vi "Read INI File.vi"(6 "Key":string, 8 "error in (no error)":errorcluster, 11 "Terminal Message in":refnum<class "Terminal Message.lvclass">) -> (0 "error out":errorcluster, 3 "Terminal Message out":refnum<class "Terminal Message.lvclass">, 4 "Message":string)   [LabVIEW 2016, in "CLD Exam - ATM.lvlib" / "Terminal Message.lvclass"]
uses:
  Terminal Message.lvclass
  Terminal Message.lvclass/Terminal Message.ctl
  <vilib>/Utility/config.llb/Read Key (String).vi
  <vilib>/Utility/config.llb/NI_LVConfig.lvlib
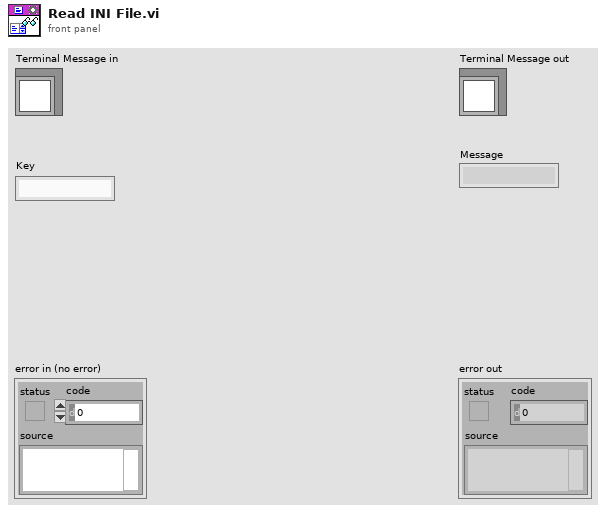
[diagram p1: front panel]
types:
  T1 = typedef "NI_LVConfig.lvlib/Config Data RefNum.ctl" = refnum<k1>
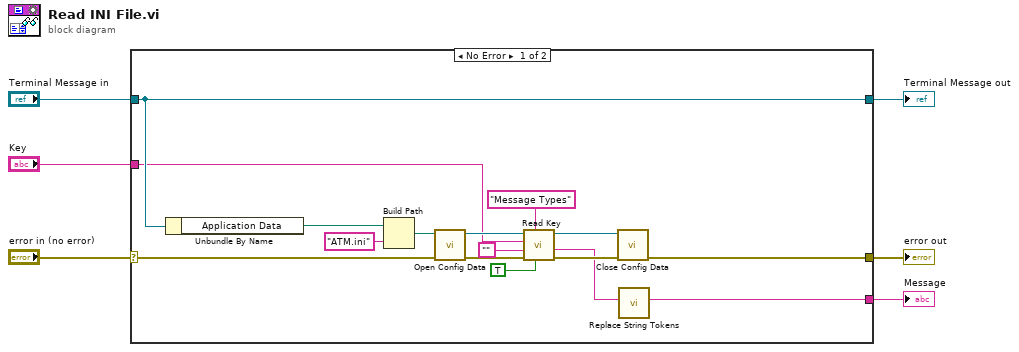
[diagram p0: block diagram]
diagram:
  n1 = case shown="No Error" "error in (no error)" {
    selector: "error in (no error)" -> [w11 w24]
    tunnel: [w12 w24] -> w5
    tunnel: [w8 w23] -> w3
    tunnel: "Terminal Message in" -> [w8 w23]
    tunnel: "Key" -> [w7 _]
    tunnel: [w9 _] -> w1
    frame No Error {
      n2 = Unbundle By Name(w8) -> ("Application Data"=w20:path)
      n3 = Build Path(base path=w20, name or relative path="ATM.ini") -> (appended path=w22:path)
      n4 = call <vilib>:"Open Config Data.vi"("error in (no error)"=w11, "configuration file path"=w22) -> ("error out"=w17:errorcluster, "refnum"=w16:T1)  [unwired: 7 in, 1 out]
      n5 = call-poly <vilib>:"Read Key.vi"("read raw string? (F)"=TRUE, "section"="Message Types", "error in (no error)"=w17, "default value"="", "key"=w7, "refnum"=w16) -> ("error out"=w13:errorcluster, "value"=w10:string, "refnum out"=w14:T1)  [unwired: 2 in, 1 out]
      n6 = call <vilib>:"Close Config Data.vi"("error in (no error)"=w13, "refnum"=w14) -> ("error out"=w12:errorcluster)  [unwired: 8 in, 1 out]
      n7 = call "Replace String Tokens.vi"("String"=w10) -> ("String out"=w9:string)  [unwired: 10 in]
    }
    frame Error {
    }
  }
  "error out" <- w5
  "Terminal Message out" <- w3
  "Message" <- w1
